vi "array to data tester.vi"() -> ()   [LabVIEW 2021]
uses:
  pdw.ctl
  mode_type.ctl
panel:
  in  "stop":bool
  in  "Cluster 2":T1
  out "Cluster":T1={"PW"=0, "frequency shift"=0.0, "amp"=0.9999923706054688, "mode type"=enum."CW", "mode depth"=0, "mode filter"=0, "phase shift"=0.0, "pulse shape filter"=0}
  # "fail at the end ??"
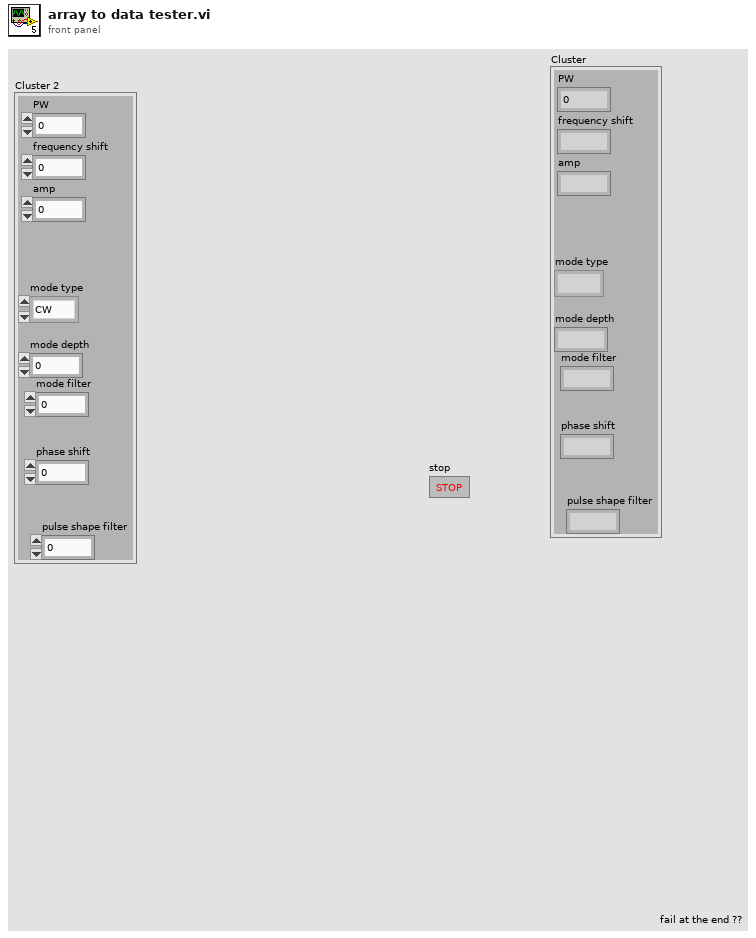
[diagram p1: front panel]
types:
  T1 = typedef "pdw.ctl" = cluster{"PW":u32, "frequency shift":fxp<+/-,48,0>, "amp":fxp<+/-,18,1>, "mode type":T2, "mode depth":u32, "mode filter":u8, "phase shift":fxp<+/-,16,1>, "pulse shape filter":u8}
  T2 = typedef "mode_type.ctl" = enum8{"CW", "NC - CW", "NC - cw", "LFM", "BPSK", "QPSK"}
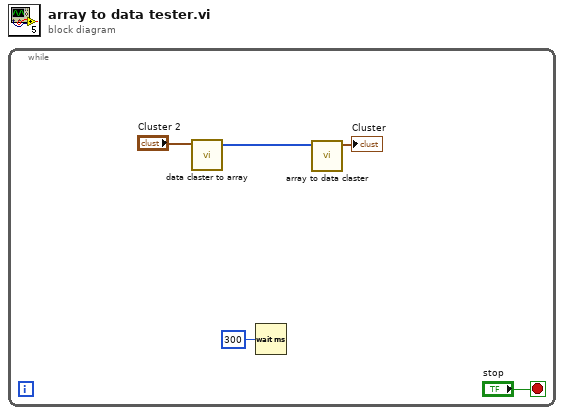
[diagram p0: block diagram]
diagram:
  n1 = while {
    stop <- "stop" stop-if-true
    n2 = call "data claster to array.vi"("Cluster"="Cluster 2") -> ("Array"=w2:u64[])  [unwired: 10 in]
    n3 = Wait (ms)(milliseconds to wait=u32 300) -> ()  [unwired: 1 out]
    n4 = call "array to data claster.vi"("Array"=w2) -> ("Cluster"=→"Cluster":T1)  [unwired: 10 in]
  }
